vi "Read Device Identification.vi"(6 "timeout ms (1000)":i32=1000, 8 "error in (no error)":errorcluster, 10 "Conformity Level":enum8{"None", "Basic", "Regular", "Extended"}(ring)=enum."Regular", 11 "Modbus TCP Micro Master in":refnum<class "Modbus TCP Micro Master.lvclass">) -> (0 "error out":errorcluster, 1 "Regular Data":T1, 2 "Objects":T2(array[cluster]), 3 "Modbus TCP Micro Master out":refnum<class "Modbus TCP Micro Master.lvclass">)   [LabVIEW 2023, in "Modbus TCP Micro.lvlib" / "Modbus TCP Micro Master.lvclass"]
uses:
  Modbus TCP Micro Master.lvclass
  Modbus TCP Micro Master.lvclass/Modbus TCP Micro Master.ctl
  Modbus TCP Micro.lvlib
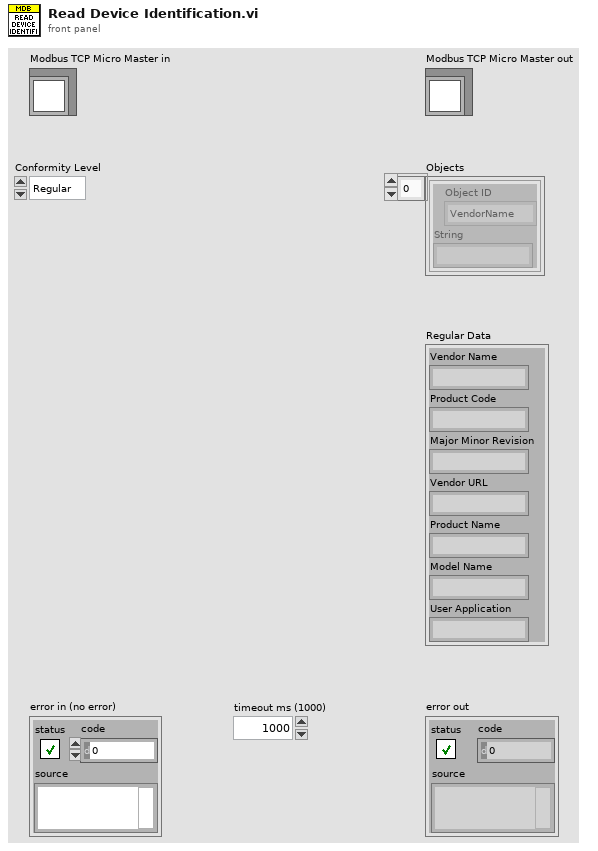
[diagram p1: front panel]
types:
  T1 = cluster{"Vendor Name":string, "Product Code":string, "Major Minor Revision":string, "Vendor URL":string, "Product Name":string, "Model Name":string, "User Application":string}
  T2 = cluster{"Object ID":enum8{"VendorName", "ProductCode", "MajorMinorRevision", "VendorUrl", "ProductName", "ModelName", "UserApplicationName"}, "String":string}[]
  T3 = enum8{"VendorName", "ProductCode", "MajorMinorRevision", "VendorUrl", "ProductName", "ModelName", "UserApplicationName"}[]
  T4 = map{enum8{"VendorName", "ProductCode", "MajorMinorRevision", "VendorUrl", "ProductName", "ModelName", "UserApplicationName"}, string}
  T5 = enum8{"VendorName", "ProductCode", "MajorMinorRevision", "VendorUrl", "ProductName", "ModelName", "UserApplicationName"}
  T6 = cluster{"[0]":string, "[1]":string, "[2]":string, "[3]":string, "[4]":string, "[5]":string, "[6]":string}
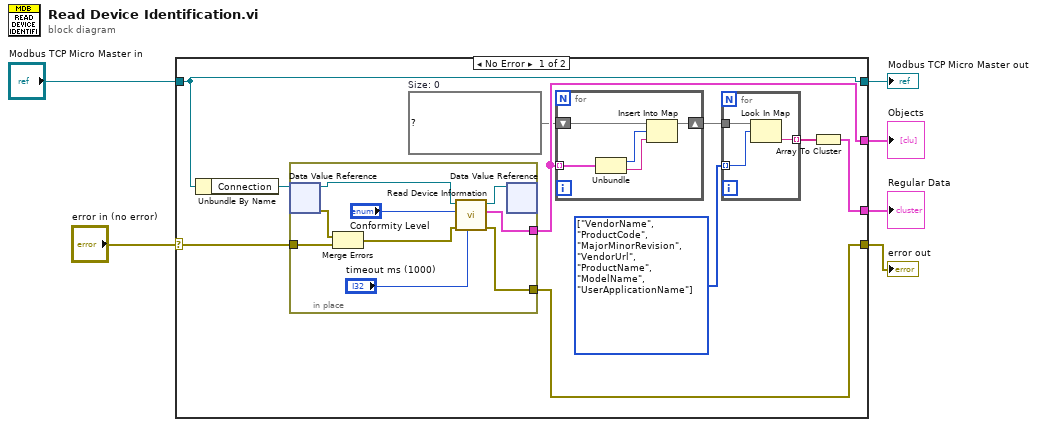
[diagram p0: block diagram]
diagram:
  n1 = case shown="No Error" "error in (no error)" {
    selector: "error in (no error)" -> [w14 w35]
    tunnel: [w13 w35] -> w5
    tunnel: [w16 w34] -> w3
    tunnel: "Modbus TCP Micro Master in" -> [w16 w34]
    tunnel: [w12 _] -> w2
    tunnel: [w7 _] -> w1
    frame No Error {
      w9 = T3 [enum."VendorName", enum."ProductCode", enum."MajorMinorRevision", enum."VendorUrl", enum."ProductName", enum."ModelName", enum."UserApplicationName"] items=["VendorName", "ProductCode", "MajorMinorRevision", "VendorUrl", "ProductName", "ModelName", "UserApplicationName"] ("Object ID")
      w11 = T4 {}  # Size: 0
      n2 = Unbundle By Name(w16) -> ("Connection"=w15:refnum<data-value>)
      n3 = in-place {
        in-place-border: w14 -> [w33]
        in-place-border: [w32] -> w13
        in-place-border: [w31] -> w12
        n4 = in-place-dvr #1(w15) -> (w30:refnum<k5>, w26:errorcluster)
        n5 = Merge Errors(w26, w33) -> (w27:errorcluster)
        n6 = call "Read Device Information.vi"("timeout ms (1000)"="timeout ms (1000)", "error in (no error)"=w27, "Conformity Level"="Conformity Level", "TCP Network Connection in"=w30) -> ("error in (no error) 2"=w32:errorcluster, "Objects"=w31:T2, "TCP Network Connection out"=w29:refnum<k5>)  [unwired: 5 in]
        n7 = in-place-dvr #1(w29) -> ()  [unwired: 2 out]
      }
      n8 = for {
        tunnel: w12 -> [w24] mode=indexing
        shift-right: [w21] -> w10
        shift-left: w11 -> [w20]
        n9 = Unbundle(w24) -> ("Object ID"=w23:T5, "String"=w22:string)
        n10 = Insert Into Map(map in=w20, key=w23, value=w22) -> (map out=w21:T4)  [unwired: 2 out]
      }
      n11 = for {
        tunnel: w10 -> [w19]
        tunnel: w9 -> [w18] mode=indexing
        tunnel: [w17] -> w8 mode=indexing
        n12 = Look In Map(map=w19, key=w18) -> (value=w17:string)  [unwired: 1 in, 1 out]
      }
      n13 = Array To Cluster(array=w8) -> (cluster=w7:T6)
    }
    frame Error {
    }
  }
  "error out" <- w5
  "Modbus TCP Micro Master out" <- w3
  "Objects" <- w2
  "Regular Data" <- w1
